vi "LCD Custom Char.vi"() -> ()   [LabVIEW 2011]
uses:
  Private/Type Defs/LCD Pin Config 4-bit.ctl
  Private/Type Defs/Chipkit Configuration.ctl
  Private/Type Defs/Board Type.ctl
  Private/Type Defs/LCD Character.ctl
  Private/Type Defs/LCD Char Row.ctl
  LabVIEW Interface for ChipKit.lvlib
panel:
  in  "LCD Character":T1
  out "LCD Character":T1
  in  "ChipKit Configuration":T3={"COM Port"="COM4", "Board Type"=enum."ChipKit uC32"}
  in  "LCD Pin Config 4 Bit":T5={"RS"=11, "RW"=255, "Enable"=9, "D4"=8, "D5"=7, "D6"=6, "D7"=5}
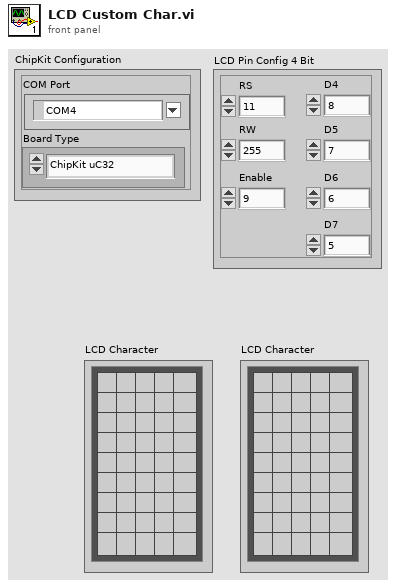
[diagram p1: front panel]
types:
  T1 = typedef "LabVIEW Interface for ChipKit.lvlib/LCD Character.ctl" = cluster{"Row 0":T2, "Row 1":T2, "Row 2":T2, "Row 3":T2, "Row 4":T2, "Row 5":T2, "Row 6":T2, "Row 7":T2, "Row 8":T2}
  T2 = typedef "LabVIEW Interface for ChipKit.lvlib/LCD Char Row.ctl" = cluster{"0":bool, "1":bool, "2":bool, "3":bool, "4":bool}
  T3 = typedef "LabVIEW Interface for ChipKit.lvlib/Chipkit Configuration.ctl" = cluster{"COM Port":refnum<visa-resource-name>, "Board Type":T4}
  T4 = typedef "LabVIEW Interface for ChipKit.lvlib/Board Type.ctl" = enum16{"ChipKit uC32", "ChipKit Uno32", "ChipKit Max32"}
  T5 = typedef "LabVIEW Interface for ChipKit.lvlib/LCD Pin Config 4-bit.ctl" = cluster{"RS":u8, "RW":u8, "Enable":u8, "D4":u8, "D5":u8, "D6":u8, "D7":u8}
  T6 = typedef "LabVIEW Interface for ChipKit.lvlib/Chipkit Resource.ctl" = cluster{"COM Port":refnum<visa-resource-name>, "Board Type":T4, "Connection Type":T7, "Baud Rate (115200)":u32, "Bytes Per Packet (15)":u32, "DI Port Num Pins":i32, "DO Port Num Pins":i32}
  T7 = typedef "LabVIEW Interface for ChipKit.lvlib/Connection Type.ctl" = enum8{"USB / Serial", "XBEE", "BlueSmirf (Bluetooth)"}
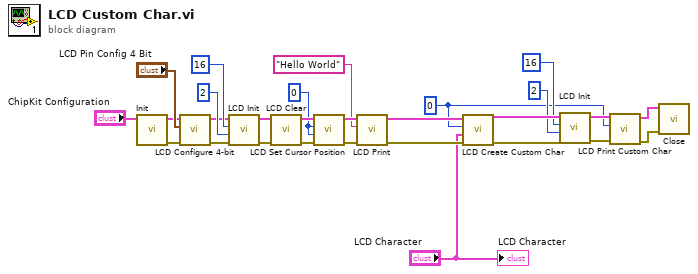
[diagram p0: block diagram]
diagram:
  w1 = u8 0 ("Custom Char Number")
  w16 = u8 0 ("Column")
  n1 = call "Init.vi"("ChipKit Configuration"="ChipKit Configuration") -> ("Error Out"=w25:errorcluster, "ChipKit Configuration"=w26:T6)  [unwired: 9 in]
  n2 = call "LCD Configure 4-bit.vi"("Error In"=w25, "LCD Pin Config 4 Bit"="LCD Pin Config 4 Bit", "ChipKit Resource"=w26) -> ("Error Out"=w22:errorcluster, "ChipKit Resource"=w21:T6)  [unwired: 7 in]
  n3 = call "LCD Init.vi"("Error In"=w22, "Rows"=u8 2, "Columns"=u8 16, "ChipKit Resource"=w21) -> ("Error Out"=w20:errorcluster, "ChipKit Resource"=w19:T6)  [unwired: 6 in]
  n4 = call "LCD Clear.vi"("Error In"=w20, "ChipKit Resource"=w19) -> ("Error Out"=w18:errorcluster, "ChipKit Resource"=w17:T6)  [unwired: 8 in]
  n5 = call "LCD Set Cursor Position.vi"("Error In"=w18, "Row"=w16, "Column"=w16, "ChipKit Resource"=w17) -> ("Error Out"=w14:errorcluster, "ChipKit Resource"=w15:T6)  [unwired: 6 in]
  n6 = call "LCD Print.vi"("Error In"=w14, "Data"="Hello World", "ChipKit Resource"=w15) -> ("Error Out"=w11:errorcluster, "ChipKit Resource"=w12:T6)  [unwired: 7 in]
  n7 = call "LCD Create Custom Char.vi"("Error In"=w11, "LCD Character"="LCD Character", "Custom Char Number"=w1, "ChipKit Resource"=w12) -> ("Error Out"=w9:errorcluster, "ChipKit Resource"=w10:T6)  [unwired: 6 in]
  n8 = call "LCD Init.vi"("Error In"=w9, "Rows"=u8 2, "Columns"=u8 16, "ChipKit Resource"=w10) -> ("Error Out"=w5:errorcluster, "ChipKit Resource"=w4:T6)  [unwired: 6 in]
  n9 = call "LCD Print Custom Char.vi"("Error In"=w5, "Custom Char Number"=w1, "ChipKit Resource"=w4) -> ("Error Out"=w2:errorcluster, "ChipKit Resource"=w3:T6)  [unwired: 7 in]
  n10 = call "Close.vi"("Error In"=w2, "ChipKit Configuration"=w3) -> ()  [unwired: 9 in, 1 out]
  "LCD Character" <- "LCD Character"
